vi "alarm_log_event_driven.vi"() -> ()   [LabVIEW 2011]
uses:
  Controls Win/enum_alarm_log.ctl
  <vilib>/Utility/file.llb/Write To Spreadsheet File (string).vi
panel:
  in  "stop":bool
  in  "Select an alarm:":u16(ring) items=["No error", "DI0", "DI1", "DI2", "DI3", "DI4", "DI5", "DI6", "DI7", "DI8", "DI9", "DI10", "DI11", "DI12", "DI13", "Input Coming from Aging Control Loop", "DI16"]
  in  "Stop Temp Exceeded":bool
  out "Temperature Exceeded:":bool
  in  "TC1:":dbl
  in  "TC0:":dbl
  in  "DI16:":bool
  in  "TC14:":dbl
  in  "DI17:":bool
  in  "Stop Standby":bool
  out "Standby:":bool
  in  "Stop Cool Down Loop":bool
  out "System Cool Down Loop:":bool
  out "Acknowledge\nManual Hard Alarm":bool
  out "System Alarm":bool
  in  "Trigger":bool
  in  "Purge System":bool
  in  "Soft Alarm Acknowledge":bool
  in  "Clear Log":bool
  out "Table":string[][](table)
  # "Alarm Log"
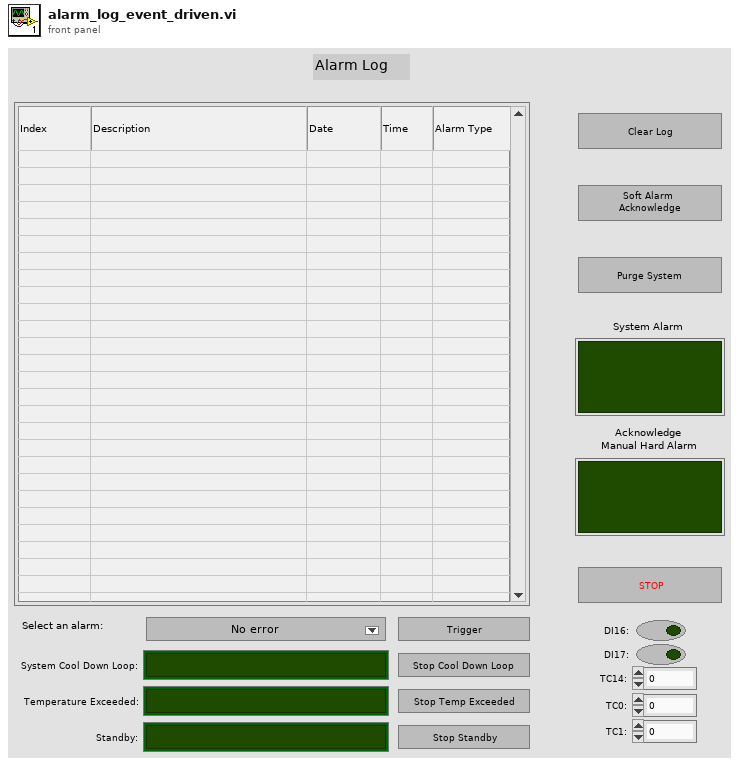
[diagram p1: front panel]
types:
  T1 = typedef "enum_alarm_log.ctl" = enum16{"do nothing", "trigger alarm", "timer elapsed", "stop temp exceeded", "thermocouple error", "clear log", "stop cool down loop", "stop standby", "soft alarm acknowledge"}
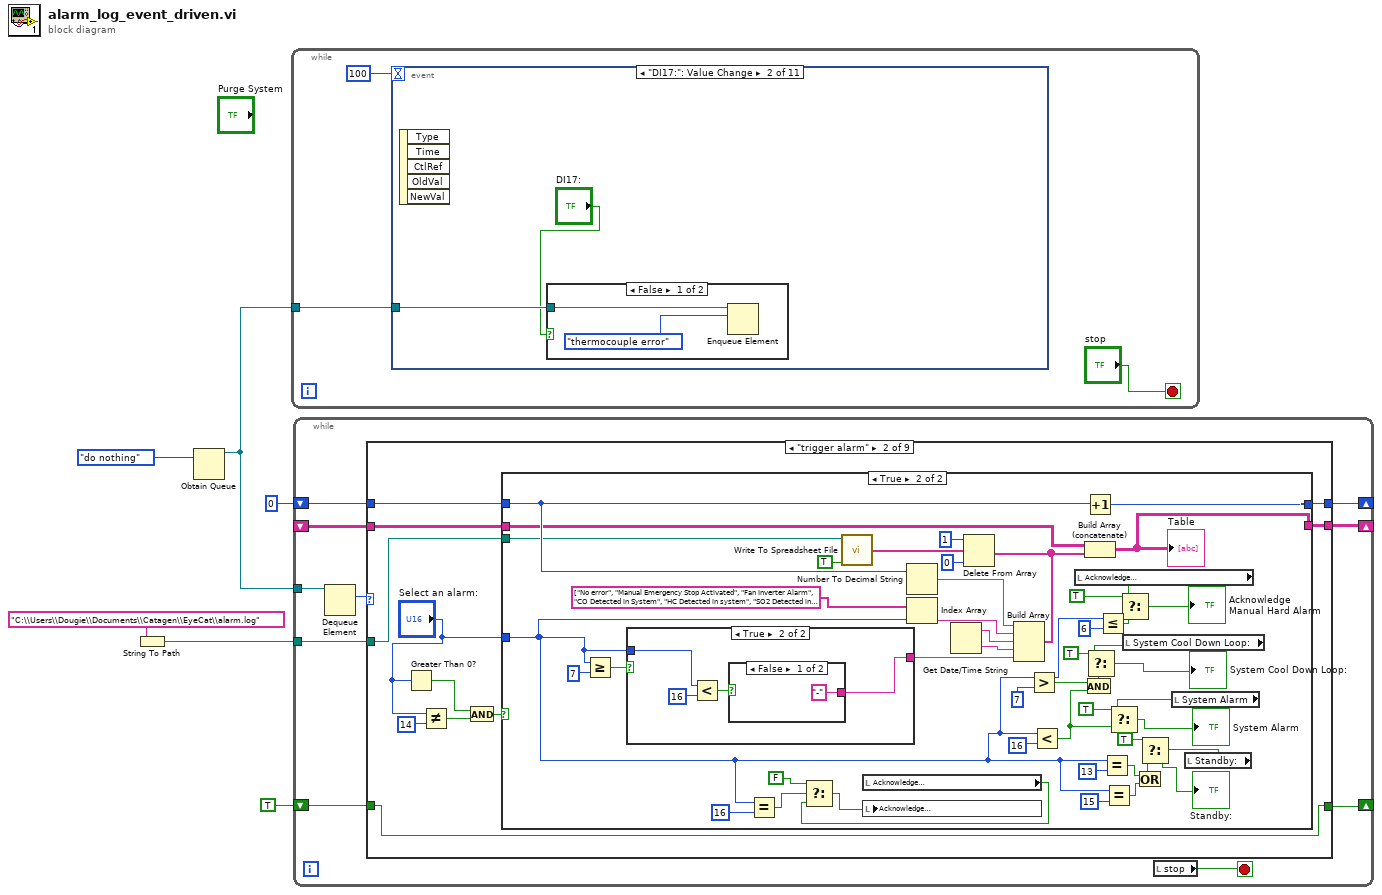
[diagram p0: block diagram]
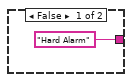
[diagram p4: hidden frame]
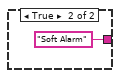
[diagram p5: hidden frame]
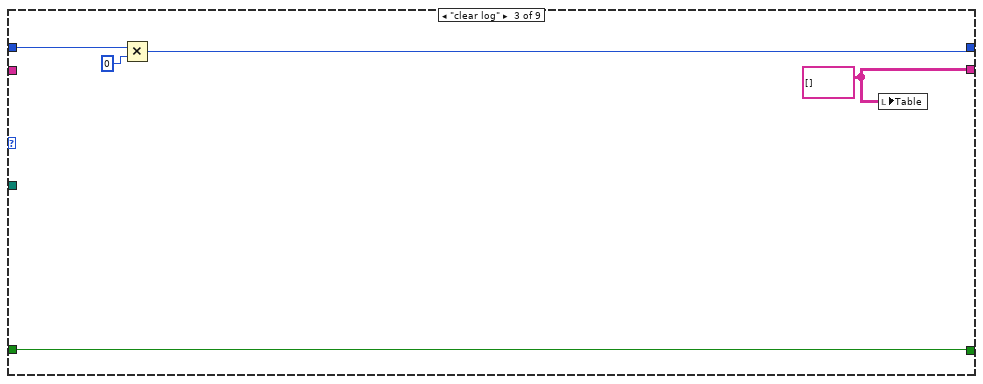
[diagram p6: hidden frame]
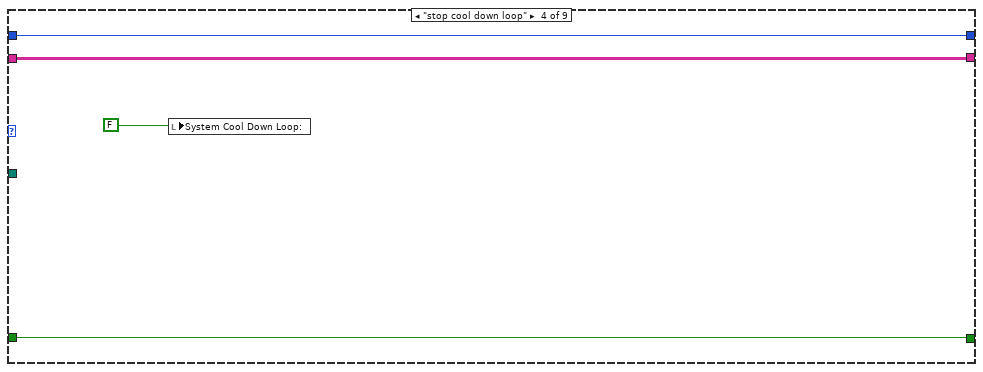
[diagram p7: hidden frame]
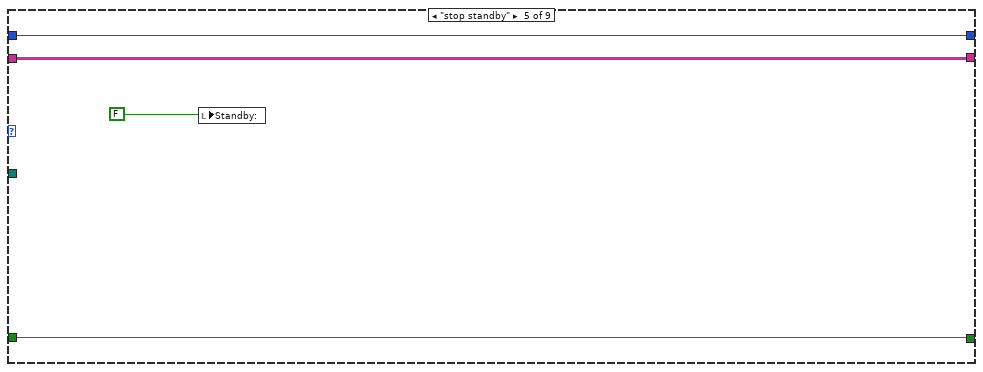
[diagram p8: hidden frame]
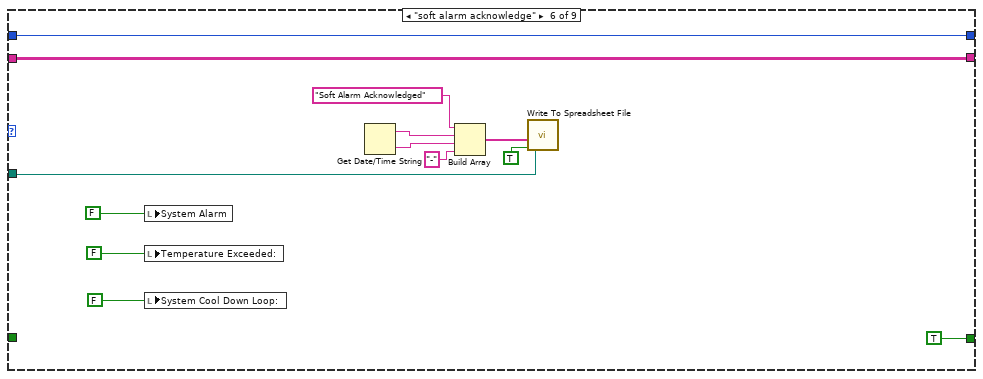
[diagram p9: hidden frame]
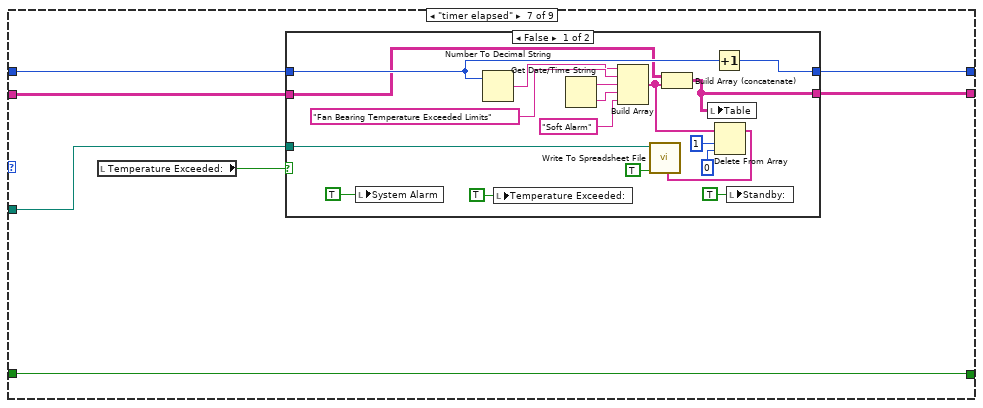
[diagram p10: hidden frame]
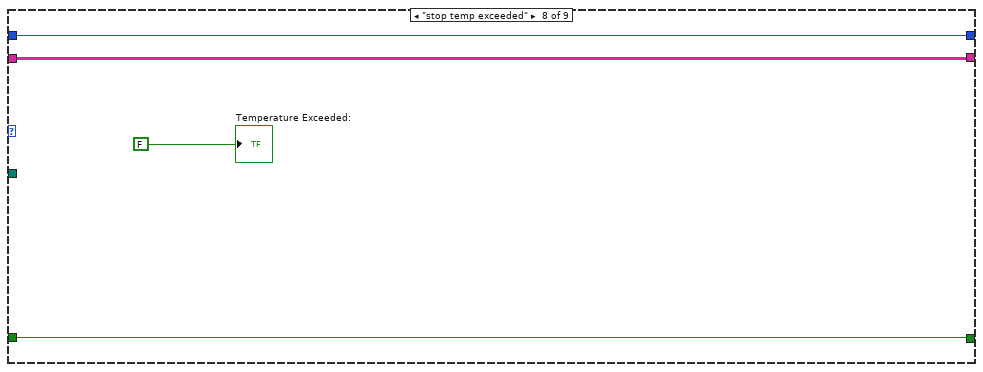
[diagram p12: hidden frame]
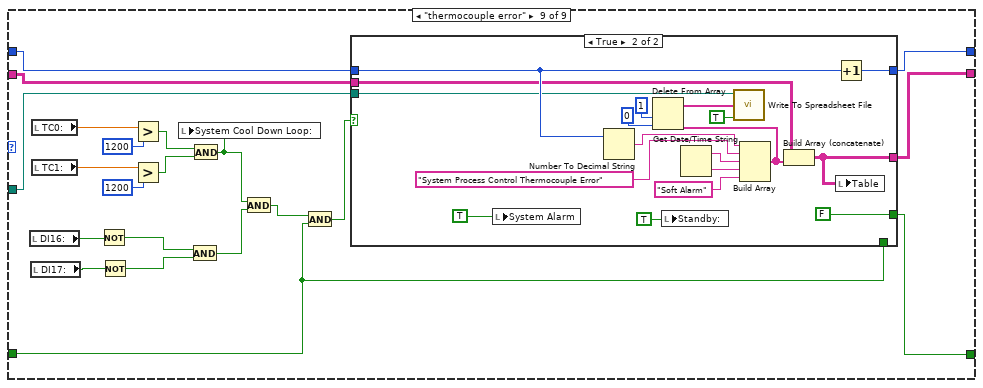
[diagram p13: hidden frame]
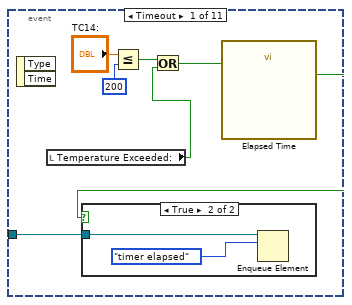
[diagram p15: hidden frame]
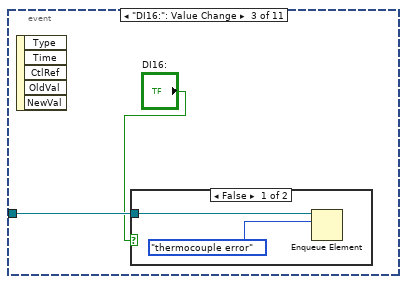
[diagram p18: hidden frame]
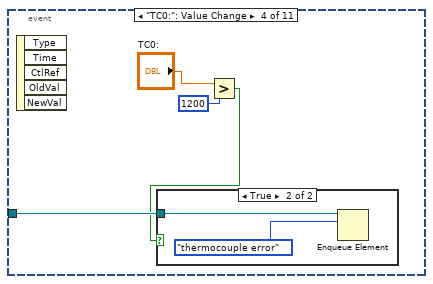
[diagram p20: hidden frame]
diagram:
  n1 = String To Path(string="C:\\Users\\Dougie\\Documents\\Catagen\\EyeCat\\alarm.log") -> (path=w1:path)
  n2 = Obtain Queue(element data type=enum_alarm_log."do nothing") -> (queue out=w5:refnum<queue>)  [unwired: 4 in, 2 out]
  n3 = while {
    tunnel: w5 -> [w8]
    stop <- "stop" stop-if-true
    n4 = event shown="[1] \"DI17:\": Value Change" {
      selector: _ -> [_ _ _ _ _ _ _ _ _ _ _]
      dyn-events: _ -> [_ _ _ _ _ _ _ _ _ _ _]
      timeout: 100 -> [_ _ _ _ _ _ _ _ _ _ _]
      tunnel: w8 -> [w15 w20 w24 w30 w36 w40 w42 w44 w46 w48 w50]
      event Timeout {
        n5 = event-data() -> ()  [unwired: 1 in, 2 out]
        n6 = local read "Temperature Exceeded:"() -> (w11:bool)
        n7 = Less Or Equal?(x="TC14:", y=200) -> (x <= y?=w12:bool)
        n8 = Or(x=w12, y=w11) -> (x .or. y?=w10:bool)
        n9 = call "Elapsed Time"("Reset"=w10) -> ("Time has Elapsed"=w13:bool)  [unwired: 11 in, 7 out]
        n10 = case shown="True" w13 {
          tunnel: w15 -> [_ w18]
          frame False {
          }
          frame True {
            n11 = Enqueue Element(queue=w18, element=enum_alarm_log."timer elapsed") -> ()  [unwired: 2 in, 3 out]
          }
        }
      }
      event "DI17:": Value Change {
        n12 = event-data() -> ()  [unwired: 1 in, 5 out]
        n13 = case shown="False" "DI17:" {
          tunnel: w20 -> [w21 _]
          frame False {
            n14 = Enqueue Element(queue=w21, element=enum_alarm_log."thermocouple error") -> ()  [unwired: 2 in, 3 out]
          }
          frame True {
          }
        }
      }
      event "DI16:": Value Change {
        n15 = event-data() -> ()  [unwired: 1 in, 5 out]
        n16 = case shown="False" "DI16:" {
          tunnel: w24 -> [w25 _]
          frame False {
            n17 = Enqueue Element(queue=w25, element=enum_alarm_log."thermocouple error") -> ()  [unwired: 2 in, 3 out]
          }
          frame True {
          }
        }
      }
      event "TC0:": Value Change {
        n18 = event-data() -> ()  [unwired: 1 in, 5 out]
        n19 = Greater?(x="TC0:", y=1200) -> (0:w27:bool)
        n20 = case shown="True" w27 {
          tunnel: w30 -> [_ w31]
          frame False {
          }
          frame True {
            n21 = Enqueue Element(queue=w31, element=enum_alarm_log."thermocouple error") -> ()  [unwired: 2 in, 3 out]
          }
        }
      }
      event "TC1:": Value Change {
        n22 = event-data() -> ()  [unwired: 1 in, 5 out]
        n23 = Greater?(x="TC1:", y=1200) -> (0:w33:bool)
        n24 = case shown="True" w33 {
          tunnel: w36 -> [_ w37]
          frame False {
          }
          frame True {
            n25 = Enqueue Element(queue=w37, element=enum_alarm_log."thermocouple error") -> ()  [unwired: 2 in, 3 out]
          }
        }
      }
      event "Stop Temp Exceeded": Value Change {
        n26 = event-data() -> ()  [unwired: 1 in, 5 out]
        n27 = Enqueue Element(queue=w40, element=enum_alarm_log."stop temp exceeded") -> ()  [unwired: 2 in, 3 out]
      }
      event "Trigger": Value Change {
        n28 = event-data() -> ()  [unwired: 1 in, 5 out]
        n29 = Enqueue Element(queue=w42, element=enum_alarm_log."trigger alarm") -> ()  [unwired: 2 in, 3 out]
      }
      event "Clear Log": Value Change {
        n30 = event-data() -> ()  [unwired: 1 in, 5 out]
        n31 = Enqueue Element(queue=w44, element=enum_alarm_log."clear log") -> ()  [unwired: 2 in, 3 out]
      }
      event "Stop Cool Down Loop": Value Change {
        n32 = event-data() -> ()  [unwired: 1 in, 5 out]
        n33 = Enqueue Element(queue=w46, element=enum_alarm_log."stop cool down loop") -> ()  [unwired: 2 in, 3 out]
      }
      event "Stop Standby": Value Change {
        n34 = event-data() -> ()  [unwired: 1 in, 5 out]
        n35 = Enqueue Element(queue=w48, element=enum_alarm_log."stop standby") -> ()  [unwired: 2 in, 3 out]
      }
      event "Soft Alarm Acknowledge": Value Change {
        n36 = event-data() -> ()  [unwired: 1 in, 5 out]
        n37 = Enqueue Element(queue=w50, element=enum_alarm_log."soft alarm acknowledge") -> ()  [unwired: 2 in, 3 out]
      }
    }
  }
  n38 = while {
    tunnel: w5 -> [w60]
    shift-right: [w57] -> _
    shift-left: 0 -> [w58]
    shift-right: [w56] -> _
    shift-left: _ -> [w55]
    shift-right: [w52] -> _
    shift-left: TRUE -> [w53]
    tunnel: w1 -> [w51]
    stop <- w54 stop-if-true
    n39 = Dequeue Element(queue=w60) -> (element=w59:T1)  [unwired: 2 in, 3 out]
    n40 = case shown="\"trigger alarm\"" w59 {
      tunnel: w58 -> [w63 w69 w136 w139 w144 w157 w164 w188 w197]
      tunnel: [w63 w68 w134 w139 w144 w157 w163 w188 w196] -> w57
      tunnel: [w62 w67 w133 w138 w143 w156 w161 w187 w194] -> w56
      tunnel: w55 -> [w62 w66 _ w138 w143 w156 w162 w187 w195]
      tunnel: w53 -> [w61 w65 w132 w137 w141 _ w159 w185 w191]
      tunnel: [w61 w65 w132 w137 w141 TRUE w159 w185 w190] -> w52
      tunnel: w51 -> [_ w64 _ _ _ w146 w158 _ w189]
      frame "do nothing", Default {
      }
      frame "trigger alarm" {
        n41 = Greater Than 0?(x="Select an alarm:") -> (x > 0?=w74:bool)
        n42 = Not Equal?(x="Select an alarm:", y=14) -> (x != y?=w72:bool)
        n43 = And(x=w74, y=w72) -> (x .and. y?=w71:bool)
        n44 = case shown="True" w71 {
          tunnel: "Select an alarm:" -> [_ w89]
          tunnel: w69 -> [w76 w114]
          tunnel: [w76 w113] -> w68
          tunnel: [w75 w111] -> w67
          tunnel: w66 -> [w75 w110]
          tunnel: w64 -> [_ w83]
          frame False {
          }
          frame True {
            n45 = Greater Or Equal?(x=w89, y=7) -> (x >= y?=w119:bool)
            n46 = case shown="True" w119 {
              tunnel: ["Hard Alarm" w128] -> w118
              tunnel: w89 -> [_ w126]
              frame False {
              }
              frame True {
                n47 = Less?(x=w126, y=16) -> (x < y?=w127:bool)
                n48 = case shown="False" w127 {
                  tunnel: ["-" "Soft Alarm"] -> w128
                  frame False {
                  }
                  frame True {
                  }
                }
              }
            }
            n49 = Equal?(x=w89, y=16) -> (x = y?=w87:bool)
            n50 = local read "Acknowledge\nManual Hard Alarm"() -> (w85:bool)
            n51 = Select(t=FALSE, s=w87, f=w85) -> (s? t:f=w84:bool)
            n52 = local write "Acknowledge\nManual Hard Alarm"(w84) -> ()
            n53 = Number To Decimal String(number=w114) -> (decimal integer string=w124:string)  [unwired: 1 in]
            n54 = Index Array(array=string[] ["No error", "Manual Emergency Stop Activated", "Fan Inverter Alarm", "CO Detected in System", "HC Detected in system", "SO2 Detected in System", "NO Detected in System", "Low Pressure in Air Line", "Low Pressure in NO Line", "Low Pressure in SO2 Line", "Low Pressure in HC Line", "Low Pressure in CO Line", "Low Pressure in N2 Line", "Low Pressure in CO2 Line", "\n", "Sample Bed Temperature Exceeded Specified Limits", "Hard Alarm Button Reset Pressed"], index=w89) -> (element=w123:string)
            n55 = Get Date/Time String() -> (date string=w122:string, time string=w121:string)  [unwired: 3 in]
            n56 = Build Array(w124, w123, w122, w121, w118) -> (w79:string[])
            n57 = Delete From Array(array=w79, length=1, index=0) -> (array with subset deleted=w78:string[])  [unwired: 1 out]
            n58 = call-poly <vilib>:"Write To Spreadsheet File.vi"("append to file? (new file:F)"=TRUE, "1D data"=w78, "file path (dialog if empty)"=w83) -> ()  [unwired: 5 in, 1 out]
            n59 = Greater?(x=w89, y=7) -> (0:w112:bool)
            n60 = Less?(x=w89, y=16) -> (x < y?=w97:bool)
            n61 = local read "Acknowledge\nManual Hard Alarm"() -> (w105:bool)
            n62 = And(x=w112, y=w97) -> (x .and. y?=w100:bool)
            n63 = Increment(x=w114) -> (x+1=w113:i32)
            n64 = Build Array (concatenate)(w110, w79) -> (w111:string[][])
            "Table" <- w111
            n65 = Less Or Equal?(x=w89, y=6) -> (x <= y?=w103:bool)
            n66 = Equal?(x=w89, y=13) -> (x = y?=w107:bool)
            n67 = Equal?(x=w89, y=15) -> (x = y?=w108:bool)
            n68 = Select(t=TRUE ("s"), s=w105, f=w103) -> (s? t:f=→"Acknowledge\nManual Hard Alarm":bool)
            n69 = local read "System Cool Down Loop:"() -> (w99:bool)
            n70 = Select(t=TRUE ("s"), s=w99, f=w100) -> (s? t:f=→"System Cool Down Loop:":bool)
            n71 = Or(x=w107, y=w108) -> (x .or. y?=w93:bool)
            n72 = local read "System Alarm"() -> (w98:bool)
            n73 = Select(t=TRUE ("s"), s=w98, f=w97) -> (s? t:f=→"System Alarm":bool)
            n74 = local read "Standby:"() -> (w92:bool)
            n75 = Select(t=TRUE ("s"), s=w92, f=w93) -> (s? t:f=→"Standby:":bool)
          }
        }
      }
      frame "clear log" {
        w133 = string[][] []
        n76 = Multiply(x=w136, y=0) -> (x*y=w134:i32)
        n77 = local write "Table"(w133) -> ()
      }
      frame "stop cool down loop" {
        n78 = local write "System Cool Down Loop:"(FALSE) -> ()
      }
      frame "stop standby" {
        n79 = local write "Standby:"(FALSE) -> ()
      }
      frame "soft alarm acknowledge" {
        n80 = local write "System Alarm"(FALSE) -> ()
        n81 = local write "Temperature Exceeded:"(FALSE ("Temperature Exceeded:")) -> ()
        n82 = local write "System Cool Down Loop:"(FALSE ("System Cool Down Loop:")) -> ()
        n83 = Get Date/Time String() -> (date string=w149:string, time string=w148:string)  [unwired: 3 in]
        n84 = Build Array("Soft Alarm Acknowledged", w149, w148, "-") -> (w150:string[])
        n85 = call-poly <vilib>:"Write To Spreadsheet File.vi"("append to file? (new file:F)"=TRUE, "1D data"=w150, "file path (dialog if empty)"=w146) -> ()  [unwired: 5 in, 1 out]
      }
      frame "timer elapsed" {
        n86 = local read "Temperature Exceeded:"() -> (w160:bool)
        n87 = case shown="False" w160 {
          tunnel: w164 -> [w177 w184]
          tunnel: [w176 w184] -> w163
          tunnel: w162 -> [w175 w183]
          tunnel: [w174 w183] -> w161
          tunnel: w158 -> [w169 _]
          frame False {
            n88 = local write "System Alarm"(TRUE) -> ()
            n89 = Number To Decimal String(number=w177) -> (decimal integer string=w178:string)  [unwired: 1 in]
            n90 = local write "Temperature Exceeded:"(TRUE ("Temperature Exceeded:")) -> ()
            n91 = Get Date/Time String() -> (date string=w180:string, time string=w181:string)  [unwired: 3 in]
            n92 = Build Array(w178, "Fan Bearing Temperature Exceeded Limits", w180, w181, "Soft Alarm") -> (w168:string[])
            n93 = Build Array (concatenate)(w175, w168) -> (w174:string[][])
            n94 = local write "Table"(w174) -> ()
            n95 = Increment(x=w177) -> (x+1=w176:i32)
            n96 = Delete From Array(array=w168, length=1, index=0) -> (array with subset deleted=w165:string[])  [unwired: 1 out]
            n97 = call-poly <vilib>:"Write To Spreadsheet File.vi"("append to file? (new file:F)"=TRUE, "1D data"=w165, "file path (dialog if empty)"=w169) -> ()  [unwired: 5 in, 1 out]
            n98 = local write "Standby:"(TRUE ("Standby:")) -> ()
          }
          frame True {
          }
        }
      }
      frame "stop temp exceeded" {
        "Temperature Exceeded:" <- FALSE ("Temperature Exceeded:")
      }
      frame "thermocouple error" {
        n99 = local read "DI16:"() -> (w205:bool)
        n100 = local read "DI17:"() -> (w204:bool)
        n101 = local read "TC0:"() -> (w206:dbl)
        n102 = local read "TC1:"() -> (w208:dbl)
        n103 = Not(x=w205) -> (.not. x?=w201:bool)
        n104 = Not(x=w204) -> (.not. x?=w200:bool)
        n105 = Greater?(x=w206, y=1200) -> (0:w203:bool)
        n106 = Greater?(x=w208, y=1200) -> (0:w202:bool)
        n107 = And(x=w201, y=w200) -> (x .and. y?=w199:bool)
        n108 = And(x=w203, y=w202) -> (x .and. y?=w198:bool)
        n109 = local write "System Cool Down Loop:"(w198) -> ()
        n110 = And(x=w198, y=w199) -> (x .and. y?=w193:bool)
        n111 = And(x=w193, y=w191) -> (x .and. y?=w192:bool)
        n112 = case shown="True" w192 {
          tunnel: w197 -> [w212 w225]
          tunnel: [w212 w224] -> w196
          tunnel: w195 -> [w211 w223]
          tunnel: [w211 w222] -> w194
          tunnel: [w210 FALSE] -> w190
          tunnel: w191 -> [w210 _]
          tunnel: w189 -> [_ w217]
          frame False {
          }
          frame True {
            n113 = local write "System Alarm"(TRUE) -> ()
            n114 = Number To Decimal String(number=w225) -> (decimal integer string=w230:string)  [unwired: 1 in]
            n115 = local write "Standby:"(TRUE) -> ()
            n116 = Get Date/Time String() -> (date string=w228:string, time string=w227:string)  [unwired: 3 in]
            n117 = Build Array(w230, "System Process Control Thermocouple Error", w228, w227, "Soft Alarm") -> (w214:string[])
            n118 = Delete From Array(array=w214, length=1, index=0) -> (array with subset deleted=w213:string[])  [unwired: 1 out]
            n119 = call-poly <vilib>:"Write To Spreadsheet File.vi"("append to file? (new file:F)"=TRUE, "1D data"=w213, "file path (dialog if empty)"=w217) -> ()  [unwired: 5 in, 1 out]
            n120 = Build Array (concatenate)(w223, w214) -> (w222:string[][])
            n121 = Increment(x=w225) -> (x+1=w224:i32)
            n122 = local write "Table"(w222) -> ()
          }
        }
      }
    }
    n123 = local read "stop"() -> (w54:bool)
  }
